vi "FindPicturesFolderFromRawData.vi"(11 "RawDataFile":path) -> (0 "SurreyPath?":bool, 1 "RawDataName":string, 2 "PicturesPath":path)   [LabVIEW 2022 SP3]
doc: "Finds the location of the Pictures folder for a given RawDataFile"
panel:
  # "Finds the location of the Pictures folder for a given RawDataFile"
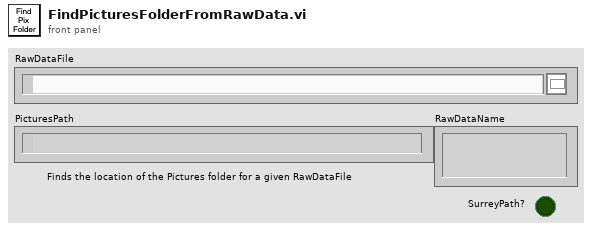
[diagram p1: front panel]
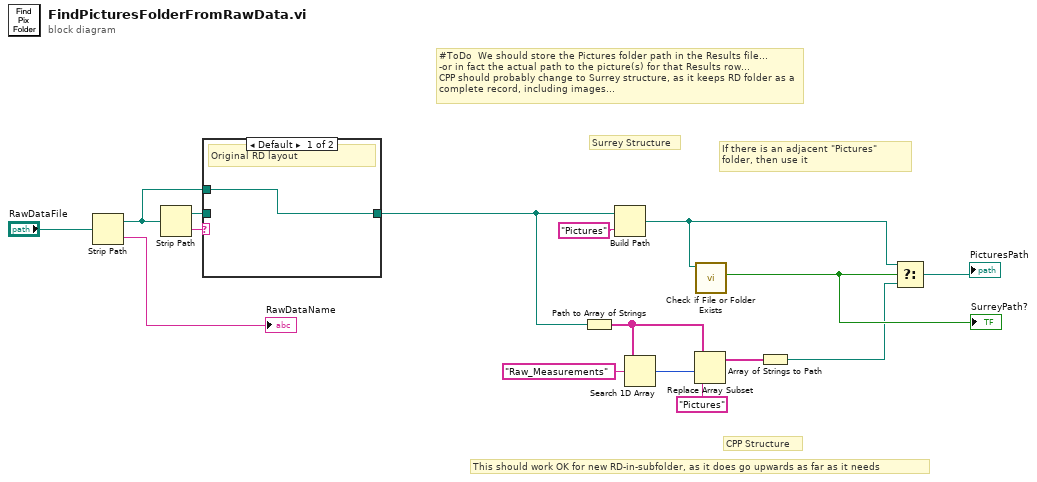
[diagram p0: block diagram]
diagram:
  # "This should work OK for new RD-in-subfolder, as it does go upwards as far as it needs"
  # "#ToDo  We should store the Pictures folder path in the Results file...\n-or in fact the actual path to the picture(s) for that Results row...\nCPP should probably change to Surrey structure, as it keeps RD folder as a complete record, including images..."
  # "If there is an adjacent \"Pictures\" folder, then use it"
  # "CPP Structure"
  # "Surrey Structure"
  n1 = Strip Path(path="RawDataFile") -> (stripped path=w1:path, name=→"RawDataName":string)
  n2 = Strip Path(path=w1) -> (stripped path=w2:path, name=w4:string)
  n3 = case shown="Default" w4 {
    tunnel: [w17 w18] -> w3
    tunnel: w2 -> [_ w18]
    tunnel: w1 -> [w17 _]
    frame Default {
      # "Original RD layout"
    }
    frame "Raw Data" {
      # "RD in subfolder"
    }
  }
  n4 = Path to Array of Strings(0:w3) -> (2:w10:string[])  [unwired: 1 out]
  n5 = Build Path(base path=w3, name or relative path="Pictures") -> (appended path=w6:path)
  n6 = Search 1D Array(1D array=w10, element="Raw_Measurements") -> (index of element=w11:i32)  [unwired: 1 in]
  n7 = Replace Array Subset(array=w10, new element="Pictures", index=w11) -> (w13:string[])
  n8 = call <vilib>:"Check if File or Folder Exists.vi"("path"=w6) -> ("file or folder exists?"=w8:bool)  [unwired: 8 in, 2 out]
  "SurreyPath?" <- w8
  n9 = Array of Strings to Path(0:w13) -> (2:w7:path)  [unwired: 1 in]
  n10 = Select(t=w6, s=w8, f=w7) -> (s? t:f=→"PicturesPath":path)
